vi "Read MICROS.vi"(8 "error in (no error)":errorcluster, 11 "SERIAL DEVICE in":refnum<class "SERIAL DEVICE.lvclass">) -> (0 "error out":errorcluster, 2 "MICROS":T1, 3 "SERIAL DEVICE out":refnum<class "SERIAL DEVICE.lvclass">)   [LabVIEW 2019, in "SERIAL DEVICE.lvclass"]
uses:
  SERIAL DEVICE.lvclass
  MICROS.ctl
  SERIAL DEVICE.lvclass/SERIAL DEVICE.ctl
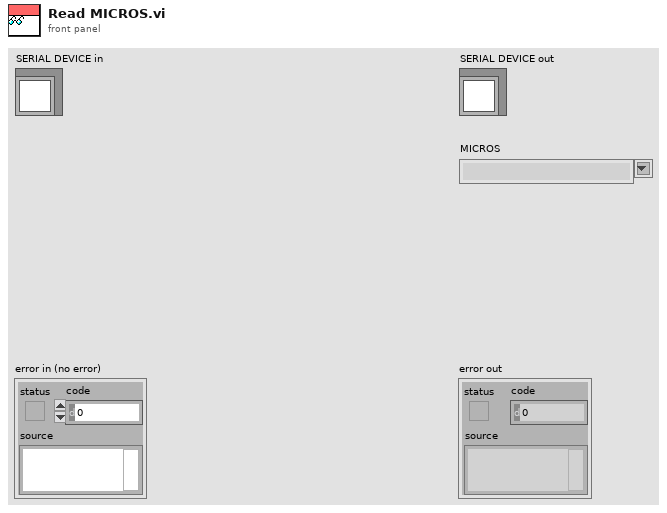
[diagram p1: front panel]
types:
  T1 = typedef "MICROS.ctl" = string
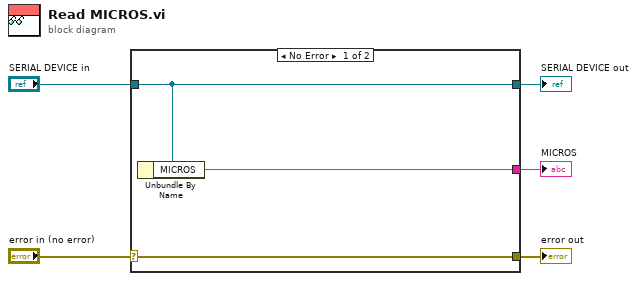
[diagram p0: block diagram]
diagram:
  n1 = case shown="No Error" "error in (no error)" {
    selector: "error in (no error)" -> [w8 w9]
    tunnel: [w8 w9] -> w4
    tunnel: [w7 w10] -> w2
    tunnel: "SERIAL DEVICE in" -> [w7 w10]
    tunnel: [w6 _] -> w1
    frame No Error {
      n2 = Unbundle By Name(w7) -> ("MICROS"=w6:T1)
    }
    frame Error {
    }
  }
  "error out" <- w4
  "SERIAL DEVICE out" <- w2
  "MICROS" <- w1
